vi "setAlignment.vi"(8 "Error In":errorcluster, 10 "alignment":T1=1 items=["AlignLeft"=1, "AlignRight"=2, "AlignHCenter"=4, "AlignJustify"=8, "AlignAbsolute"=16, "AlignHorizontal_Mask"=31, "AlignTop"=32, "AlignBottom"=64, "AlignVCenter"=128, "AlignBaseline"=256, "AlignVertical_Mask"=480, "AlignCenter"=132], 11 "QGroupBox In":refnum<class "QGroupBox.lvclass">) -> (0 "Error Out":errorcluster, 3 "QGroupBox Out":refnum<class "QGroupBox.lvclass">)   [LabVIEW 2014, in "QGroupBox.lvclass"]
doc: "LabVIEW-specific documentation is not yet available. See <b>https://doc.qt.io/qt-5/qgroupbox.html#setAlignment</b>"
uses:
  QGroupBox.lvclass
  LQ Core/Qt/AlignmentFlag.ctl
  LQ Core/LQIdentity/LQIdentity.lvclass/LQIdentity.ctl
  LQ Core/LQ Core.lvlib
  LQ Core/LQIdentity/LQIdentity.lvclass
  LQ Core/Qt/Qt.lvlib
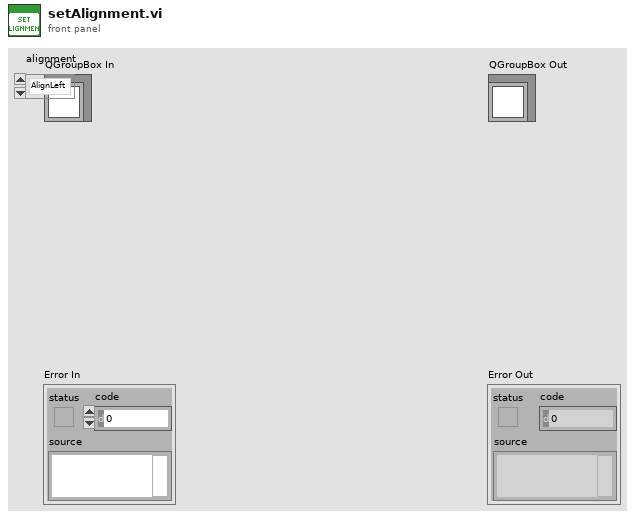
[diagram p1: front panel]
types:
  T1 = typedef "Qt.lvlib/AlignmentFlag.ctl" = i32
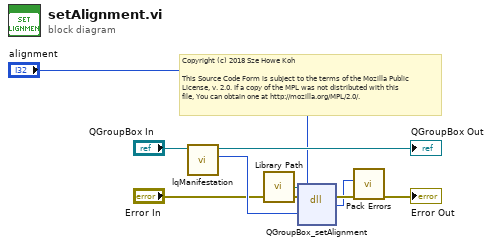
[diagram p0: block diagram]
diagram:
  # "Copyright (c) 2018 Sze Howe Koh\n\nThis Source Code Form is subject to the terms of the Mozilla Public\nLicense, v. 2.0. If a copy of the MPL was not distributed with this\nfile, You can obtain one at http://mozilla.org/MPL/2.0/."
  n1 = call "lqManifestation.vi"("LQIdentity in"="QGroupBox In") -> ("Manifestation"=w6:u64, "LQIdentity out"=→"QGroupBox Out":refnum<class "QGroupBox.lvclass">)  [unwired: 9 in]
  n2 = call "Library Path.vi"() -> ("Library Path"=w7:path)
  n3 = dll-call lib="?" fn="QGroupBox_setAlignment"(path in=w7, error in="Error In", "_instance"=w6, "alignment"="alignment") -> (error out=w4:errorcluster, w2:i32)  [unwired: 3 in, 1 out]
  n4 = call "Pack Errors.vi"("Error In"=w4, "Error Code"=w2) -> ("Error Out"=→"Error Out":errorcluster)  [unwired: 9 in]
